vi "MotorTracking.vi"   [LabVIEW 2011]
uses:
  Manual-Auto.vi
  Global 1.vi
types:
  T1 = cluster{"Position":cluster{"X":dbl, "Y":dbl}, "Distance (ft)":dbl}[]
  T2 = typedef "WPI_JoystickDevRef.ctl" = cluster{"Device":T3}
  T3 = typedef "WPI_JoystickDeviceEnum.ctl" = enum16{"USB 1", "USB 2", "USB 3", "USB 4", "Kinect 1", "Kinect 2"}
  T4 = typedef "WPI_JoystickButtonState.ctl" = cluster{"Button 1":bool, "Button 2":bool, "Button 3":bool, "Button 4":bool, "Button 5":bool, "Button 6":bool, "Button 7":bool, "Button 8":bool, "Button 9":bool, "Button 10":bool, "Button 11":bool, "Button 12":bool}
  T5 = typedef "WPI_DigitalInputDevRef.ctl" = cluster{"DevStatus":errorcluster, "DIO Channel":T6, "Digital Module":T7}
  T6 = typedef "FPGA_DIOChannel.ctl" = enum8{"DIO 1", "DIO 2", "DIO 3", "DIO 4", "DIO 5", "DIO 6", "DIO 7", "DIO 8", "DIO 9", "DIO 10", "DIO 11", "DIO 12", "DIO 13", "DIO 14", "Invalid"}
  T7 = typedef "FPGA_TypedefDigitalModule.ctl" = enum16{"Digital Module 1", "Digital Module 2"}
  T8 = cluster{"Target Info[0]":cluster{"Position":cluster{"X":dbl, "Y":dbl}, "Distance (ft)":dbl}, "Target Info[1]":cluster{"Position":cluster{"X":dbl, "Y":dbl}, "Distance (ft)":dbl}, "Target Info[2]":cluster{"Position":cluster{"X":dbl, "Y":dbl}, "Distance (ft)":dbl}, "Target Info[3]":cluster{"Position":cluster{"X":dbl, "Y":dbl}, "Distance (ft)":dbl}, "Target Info[4]":cluster{"Position":cluster{"X":dbl, "Y":dbl}, "Distance (ft)":dbl}, "Target Info[5]":cluster{"Position":cluster{"X":dbl, "Y":dbl}, "Distance (ft)":dbl}, "Target Info[6]":cluster{"Position":cluster{"X":dbl, "Y":dbl}, "Distance (ft)":dbl}, "Target Info[7]":cluster{"Position":cluster{"X":dbl, "Y":dbl}, "Distance (ft)":dbl}, "Target Info[8]":cluster{"Position":cluster{"X":dbl, "Y":dbl}, "Distance (ft)":dbl}}
  T9 = typedef "WPI_MotorControlDeviceRef.ctl" = cluster{"DeviceStatus":errorcluster, "Type":enum16{"PWM", "CAN"}, "PWM":cluster{"Digital Module":T7, "PWM Channel":T10, "DeadBand":T11}, "CAN":cluster{"Device Number":u8, "Control Mode":T12, "Semaphore":T13, "Max Vout":dbl}, "Invert":bool, "TransformRef":T14, "InvTransformRef":T14}
  T10 = typedef "FPGA_DIOPWMChannel.ctl" = enum8{"PWM 1", "PWM 2", "PWM 3", "PWM 4", "PWM 5", "PWM 6", "PWM 7", "PWM 8", "PWM 9", "PWM 10", "Invalid"}
  T11 = typedef "WPI_PWMDeadband.ctl" = cluster{"Name":string, "maxPositivePwm":i32, "minPositivePwm":i32, "centerPwm":i32, "maxNegativePwm":i32, "minNegativePwm":i32, "angularRange":u16}
  T12 = typedef "WPI_CANJaguar_ControlMode.ctl" = enum8{"Percent VBus", "Current", "Speed", "Position", "Voltage"}
  T13 = typedef "Semaphore RefNum" = refnum<k1>
  T14 = typedef "WPI_PWMTransform_ConPane.ctl" = refnum<vi>
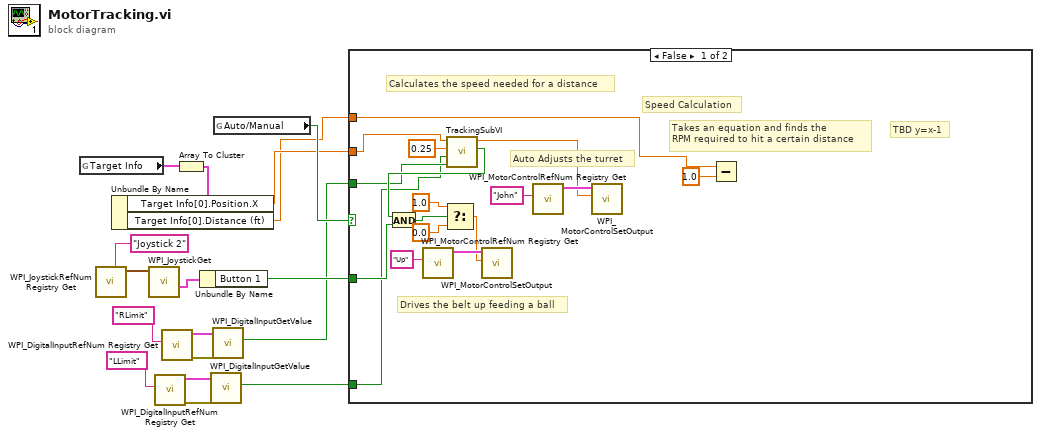
[diagram p0: block diagram]
diagram:
  n1 = global read "Global 1.vi" "Target Info"() -> (w15:T1)
  n2 = call <vilib>:"WPI_JoystickRefNum Registry Get.vi"("refnum name"="Joystick 2") -> ("JoystickDevRef"=w13:T2)  [unwired: 9 in, 1 out]
  n3 = call <vilib>:"WPI_JoystickGet.vi"("JoystickDevRef"=w13) -> ("Buttons"=w11:T4)  [unwired: 4 in, 2 out]
  n4 = call <vilib>:"WPI_DigitalInputRefNum Registry Get.vi"("refnum name"="LLimit") -> ("error out"=w6:errorcluster, "DigitalInputDevRef"=w5:T5)  [unwired: 9 in]
  n5 = call <vilib>:"WPI_DigitalInputRefNum Registry Get.vi"("refnum name"="RLimit") -> ("error out"=w9:errorcluster, "DigitalInputDevRef"=w8:T5)  [unwired: 9 in]
  n6 = Array To Cluster(array=w15) -> (cluster=w16:T8)
  n7 = Unbundle By Name(w16) -> ("Target Info[0].Position.X"=w14:dbl, "Target Info[0].Distance (ft)"=w1:dbl)
  n8 = Unbundle By Name(w11) -> ("Button 1"=w10:bool)
  n9 = call <vilib>:"WPI_DigitalInputGetValue.vi"("error in (no error)"=w6, "DigitalInputDevRef"=w5) -> ("Value"=w2:bool)  [unwired: 7 in, 2 out]
  n10 = call <vilib>:"WPI_DigitalInputGetValue.vi"("error in (no error)"=w9, "DigitalInputDevRef"=w8) -> ("Value"=w3:bool)  [unwired: 7 in, 2 out]
  n11 = global read "Manual-Auto.vi" "Auto/Manual"() -> (w17:bool)
  n12 = case shown="False" w17 {
    tunnel: w14 -> [w34 _]
    tunnel: w10 -> [w31 _]
    tunnel: w3 -> [w21 _]
    tunnel: w2 -> [w20 _]
    tunnel: w1 -> [w19 _]
    frame False {
      # "TBD y=x-1"
      # "Takes an equation and finds the\nRPM required to hit a certain distance"
      # "Speed Calculation"
      # "Auto Adjusts the turret"
      # "Drives the belt up feeding a ball"
      # "Calculates the speed needed for a distance"
      n13 = call <vilib>:"WPI_MotorControlRefNum Registry Get.vi"("refnum name"="Up") -> ("MotorControlDevRef"=w28:T9)  [unwired: 9 in, 1 out]
      n14 = call "TrackingSubVI.vi"("Right Limit"=w21, "Left Limit"=w20, "Tolerance"=0.25, "Actual Position (x)"=w34) -> ("Fire!"=w32:bool, "Motor Out"=w22:dbl)  [unwired: 6 in]
      n15 = And(x=w32, y=w31) -> (x .and. y?=w30:bool)
      n16 = Select(t=1.0, s=w30, f=0.0) -> (s? t:f=w27:dbl)
      n17 = call <vilib>:"WPI_MotorControlSetOutput.vi"("Output"=w27, "MotorControlDevRef"=w28) -> ()  [unwired: 8 in, 2 out]
      n18 = call <vilib>:"WPI_MotorControlRefNum Registry Get.vi"("refnum name"="John") -> ("MotorControlDevRef"=w23:T9)  [unwired: 9 in, 1 out]
      n19 = call <vilib>:"WPI_MotorControlSetOutput.vi"("Output"=w22, "MotorControlDevRef"=w23) -> ()  [unwired: 8 in, 2 out]
      n20 = Subtract(x=w19, y=1.0) -> ()  [unwired: 1 out]
    }
    frame True {
      # "Manual is handled in teleop. :("
      # "Takes the X value fr"
    }
  }
